vi "Baud_Set.vi"(8 "error in (no error)":errorcluster caption="错误输入（无错误）", 10 "波特率":u32, 11 "Serial输入":refnum<class "Serial.lvclass">) -> (0 "error out":errorcluster caption="错误输出", 3 "Serial输出":refnum<class "Serial.lvclass">)   [LabVIEW 2012, in "Serial.lvclass"]
uses:
  Serial.lvclass
  Serial.lvclass/Serial.ctl
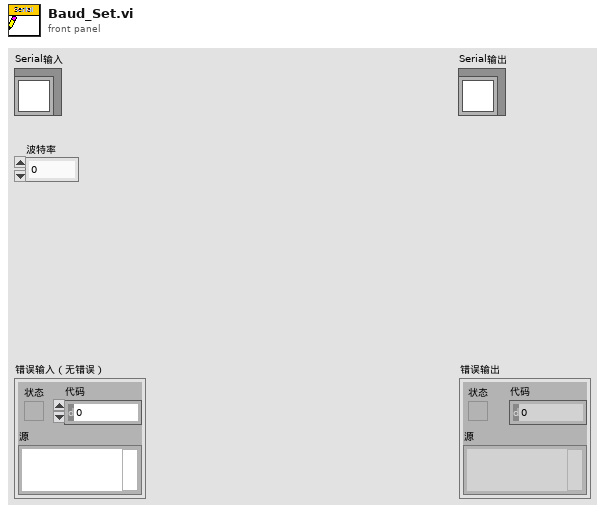
[diagram p1: front panel]
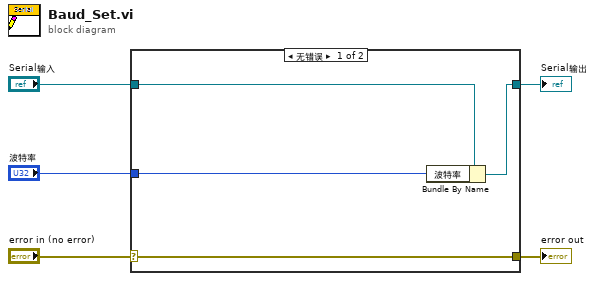
[diagram p0: block diagram]
diagram:
  n1 = case shown="无错误" "error in (no error)" {
    selector: "error in (no error)" -> [w9 w10]
    tunnel: [w9 w10] -> w4
    tunnel: [w7 w11] -> w2
    tunnel: "Serial输入" -> [w8 w11]
    tunnel: "波特率" -> [w6 _]
    frame No Error {
      n2 = Bundle By Name(cluster=w8, "波特率"=w6) -> (w7:refnum<class "Serial.lvclass">)
    }
    frame Error {
    }
  }
  "error out" <- w4
  "Serial输出" <- w2
